vi "Program28.vi"() -> ()   [LabVIEW 2020]
panel:
  out "Tablica":string[](array[string])
  out "Sciezka dostepu":path
  out "Odczytany plik":string
  out "Tekst do zapisu":string
  in  "Tekst":string
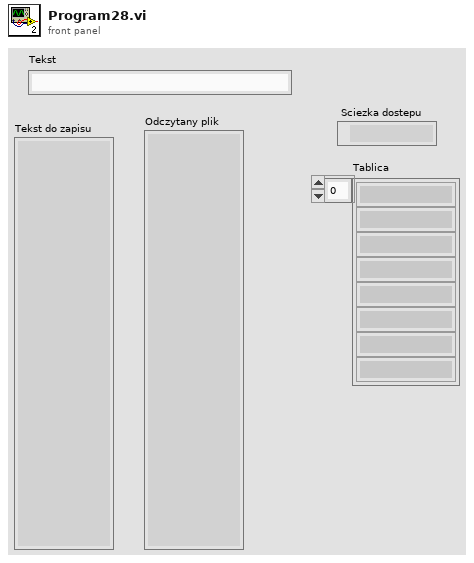
[diagram p1: front panel]
types:
  T1 = enum16{"open", "replace", "create", "open or create", "replace or create", "replace or create with confirmation"}
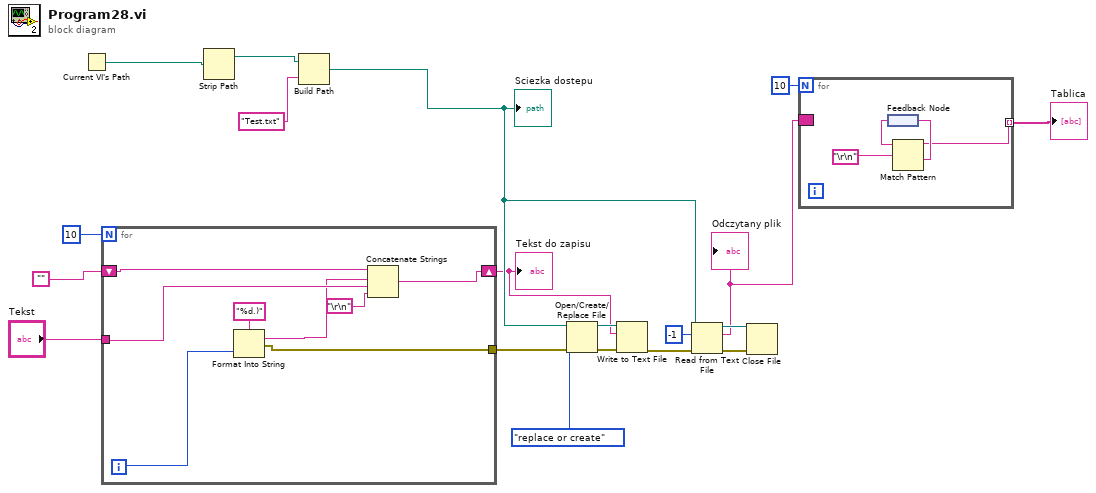
[diagram p0: block diagram]
diagram:
  n1 = Current VI's Path() -> (path=w19:path)
  n2 = for {
    N: 10 -> [_]
    shift-right: [w26] -> w1
    shift-left: "" -> [w27]
    tunnel: "Tekst" -> [w25]
    tunnel: [w20] -> w3
    i -> [w22]
    n3 = Format Into String(format string="%d.)", w22) -> (resulting string=w23:string, error out=w20:errorcluster)  [unwired: 2 in]
    n4 = Concatenate Strings(w27, w23, w25, "\r\n") -> (w26:string)
  }
  "Tekst do zapisu" <- w1
  n5 = Strip Path(path=w19) -> (stripped path=w18:path)  [unwired: 1 out]
  n6 = Build Path(base path=w18, name or relative path="Test.txt") -> (appended path=w7:path)
  "Sciezka dostepu" <- w7
  n7 = Open/Create/Replace File(file path (use dialog)=w7, error in=w3, operation (0:open)=T1."replace or create") -> (refnum out=w8:refnum<file>, error out=w13:errorcluster)  [unwired: 3 in, 1 out]
  n8 = Write to Text File(file (use dialog)=w8, text=w1, error in=w13) -> (error out=w12:errorcluster)  [unwired: 1 in, 2 out]
  n9 = Read from Text File(file (use dialog)=w7, count=-1, error in=w12) -> (refnum out=w10:refnum<file>, text=w5:string, error out=w11:errorcluster)  [unwired: 1 in, 1 out]
  "Odczytany plik" <- w5
  n10 = Close File(refnum=w10, error in=w11) -> ()  [unwired: 2 out]
  n11 = for {
    N: 10 -> [_]
    border: w5 -> [_]
    tunnel: [w30] -> w4 mode=indexing
    n12 = feedback #1() -> (w29:string)
    n13 = Match Pattern(string=w29, regular expression="\r\n") -> (before substring=w30:string, after substring=w31:string)  [unwired: 1 in, 2 out]
    n14 = feedback-in #1(w31) -> ()
  }
  "Tablica" <- w4
